vi "Delete Prompt.vi"(0 "VISA resource name":refnum<visa-resource-name>, 11 "error in (no error)":errorcluster) -> (4 "VISA resource name out":refnum<visa-resource-name>, 15 "error out":errorcluster)   [LabVIEW 2014, in "eec 6700.lvlib"]
doc: "Deletes the prompt set in the active step."
uses:
  <instrlib>/eec 6700/eec 6700.lvlib
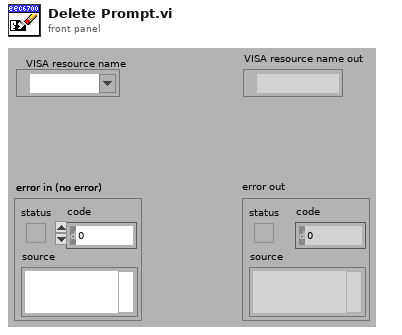
[diagram p1: front panel]
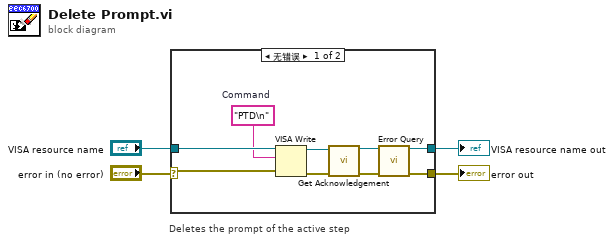
[diagram p0: block diagram]
diagram:
  # "Deletes the prompt of the active step"
  n1 = case shown="无错误" "error in (no error)" {
    selector: "error in (no error)" -> [w12 w15]
    tunnel: "VISA resource name" -> [w13 w14]
    tunnel: [w11 w14] -> w3
    tunnel: [w10 w15] -> w2
    frame No Error {
      w9 = "PTD\n"  # Command
      n2 = VISA Write(VISA resource name=w13, write buffer=w9, error in (no error)=w12) -> (VISA resource name out=w5:refnum<visa-resource-name>, error out=w6:errorcluster)  [unwired: 1 out]
      n3 = call <instrlib>:"Get Acknowledgement.vi"("VISA resource name"=w5, "error in (no error)"=w6) -> ("VISA resource name out"=w8:refnum<visa-resource-name>, "error out"=w7:errorcluster)  [unwired: 12 in]
      n4 = call <instrlib>:"Error Query.vi"("VISA resource name"=w8, "error in (no error)"=w7) -> ("VISA resource name out"=w11:refnum<visa-resource-name>, "error out"=w10:errorcluster)  [unwired: 10 in, 2 out]
    }
    frame Error {
    }
  }
  "error out" <- w2
  "VISA resource name out" <- w3
